vi "FTW-CodeGen-ChooseImplementation.vi"(0 "GObject to Traverse":refnum<vi>, 5 "Diagram Disable Structure Label":string="@FTW-CodeGen", 7 "Visible Frame":u32, 11 "error in":errorcluster) -> (15 "error out":errorcluster)   [LabVIEW 2014]
panel:
  # "Inputs"
  # "Outputs"
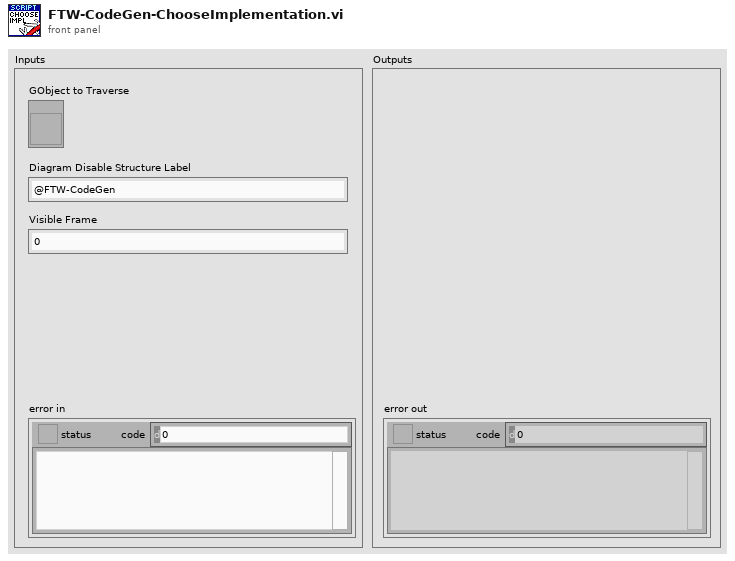
[diagram p1: front panel]
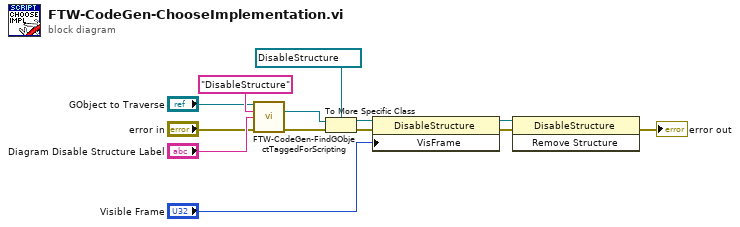
[diagram p0: block diagram]
diagram:
  n1 = call "FTW-CodeGen-FindGObjectTaggedForScripting.vi"("GObject to Traverse"="GObject to Traverse", "Class Name"="DisableStructure", "Label Prefix to uniquely identify node"="Diagram Disable Structure Label", "error in"="error in") -> ("GObject"=w12:refnum<vi>, "error out"=w11:errorcluster)  [unwired: 10 in]
  n2 = To More Specific Class(target class=refnum<vi> refnum ("Object"), reference=w12, error in=w11) -> (specific class reference=w10:refnum<vi>, error out=w9:errorcluster)
  n3 = property class="DisableStructure"(reference=w10, error in=w9, "VisFrame"="Visible Frame") -> (reference out=w4:refnum<vi>, error out=w2:errorcluster)
  n4 = invoke class="DisableStructure" method="Remove Structure"(reference=w4, error in=w2) -> (error out=→"error out":errorcluster)  [unwired: 1 in, 2 out]
